vi "display queue.vi"(7 "Action":T1=enum."Enqueue", 8 "error in (no error)":errorcluster, 9 "max queue size (-1, unlimited)":i32=1, 10 "time out":i32=100, 11 "input data":u16[](array[numeric])) -> (0 "error out":errorcluster, 1 "timed out?":bool, 2 "Empty?":bool, 3 "output data":u16[](array[numeric]), 5 "# elements in queue":i32)   [LabVIEW 2018]
uses:
  Controls/Queue Manager Actions.ctl
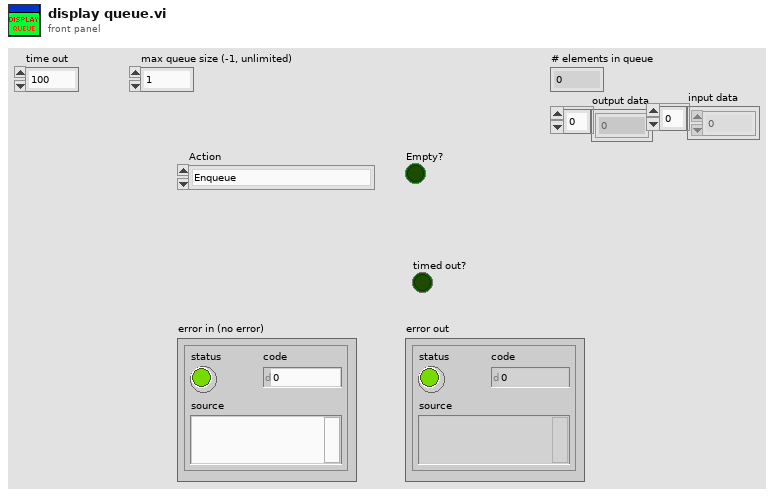
[diagram p1: front panel]
types:
  T1 = typedef "Queue Manager Actions.ctl" = enum16{"Init", "Enqueue", "Enqueue All", "Preview Queue", "Dequeue", "Get Status", "Flush Queue", "Flush All Queues", "Release All Queues", "Release Queue", "Enqueue at Opposite End"}
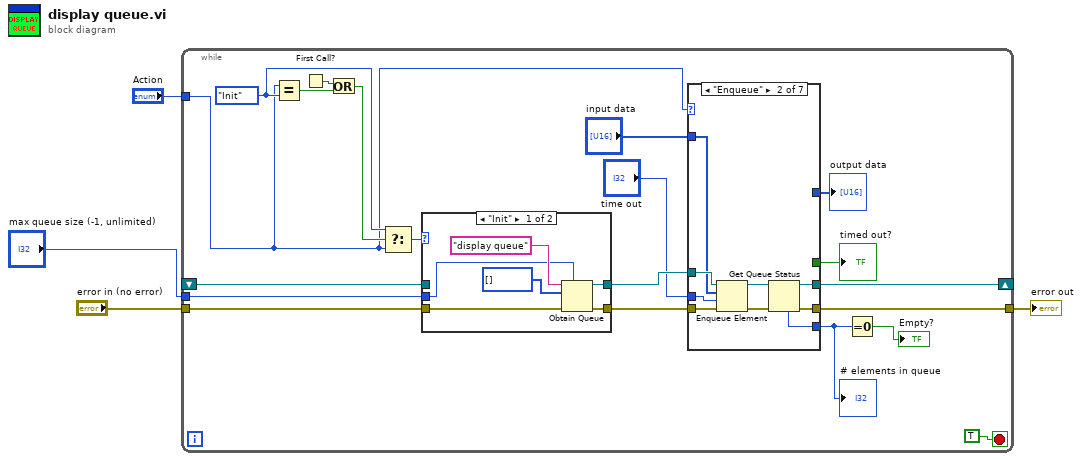
[diagram p0: block diagram]
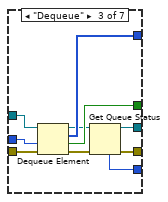
[diagram p3: hidden frame]
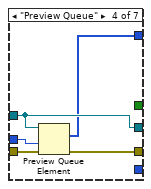
[diagram p4: hidden frame]
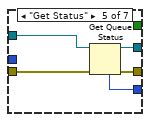
[diagram p5: hidden frame]
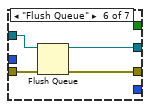
[diagram p6: hidden frame]
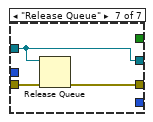
[diagram p7: hidden frame]
diagram:
  n1 = while {
    tunnel: "Action" -> [w12]
    tunnel: "error in (no error)" -> [w19]
    tunnel: [w18] -> w2
    shift-right: [w14] -> _
    shift-left: _ -> [w13]
    tunnel: "max queue size (-1, unlimited)" -> [w7]
    stop <- TRUE stop-if-true
    w21 = Queue_Manager_Actions."Init"
    n2 = Equal?(x=w12, y=w21) -> (x = y?=w23:bool)
    n3 = First Call?() -> (First Call?: T/F=w24:bool)
    n4 = Or(x=w24, y=w23) -> (x .or. y?=w22:bool)
    n5 = Select(t=w21, s=w22, f=w12) -> (s? t:f=w20:T1)
    n6 = case shown="\"Init\"" w20 {
      tunnel: [w68 w69] -> w16
      tunnel: w19 -> [w67 w70]
      tunnel: [w66 w70] -> w17
      tunnel: w13 -> [_ w69]
      tunnel: w7 -> [w63 _]
      frame "Init" {
        n7 = Obtain Queue(max queue size (-1, unlimited)=w63, name (unnamed)="display queue" ("queue name"), element data type=u16[] [], error in (no error)=w67) -> (queue out=w68:refnum<queue>, error out=w66:errorcluster)  [unwired: 1 in, 1 out]
      }
      frame "Enqueue", Default {
      }
    }
    n8 = case shown="\"Enqueue\"" w12 {
      tunnel: w16 -> [w25 w33 w43 w47 w53 w57 w60]
      tunnel: [w26 w29 w39 w49 w54 w58 w61] -> w18
      tunnel: w17 -> [w26 w35 w45 w50 w55 w59 w62]
      tunnel: [w25 w31 w38 w47 w52 w56 w60] -> w14
      tunnel: "time out" -> [_ w34 w44 w48 _ _ _]
      tunnel: [_ w28 w36 _ w51 _ _] -> w10
      tunnel: [_ _ w42 w46 _ _ _] -> w6
      tunnel: [_ _ w41 _ _ _ _] -> w9
      tunnel: "input data" -> [_ w27 _ _ _ _ _]
      frame "Init", Default {
      }
      frame "Enqueue" {
        n9 = Enqueue Element(queue=w33, element=w27, timeout in ms (-1)=w34, error in (no error)=w35) -> (queue out=w32:refnum<queue>, error out=w30:errorcluster)  [unwired: 1 out]
        n10 = Get Queue Status(queue=w32, error in (no error)=w30) -> (queue out=w31:refnum<queue>, error out=w29:errorcluster, # elements in queue=w28:i32)  [unwired: 1 in, 5 out]
      }
      frame "Dequeue" {
        n11 = Dequeue Element(queue=w43, timeout in ms (-1)=w44, error in (no error)=w45) -> (queue out=w37:refnum<queue>, element=w42:u16[], timed out?=w41:bool, error out=w40:errorcluster)
        n12 = Get Queue Status(queue=w37, error in (no error)=w40) -> (queue out=w38:refnum<queue>, error out=w39:errorcluster, # elements in queue=w36:i32)  [unwired: 1 in, 5 out]
      }
      frame "Preview Queue" {
        n13 = Preview Queue Element(queue=w47, timeout in ms (-1)=w48, error in (no error)=w50) -> (element=w46:u16[], error out=w49:errorcluster)  [unwired: 2 out]
      }
      frame "Get Status" {
        n14 = Get Queue Status(queue=w53, error in (no error)=w55) -> (queue out=w52:refnum<queue>, error out=w54:errorcluster, # elements in queue=w51:i32)  [unwired: 1 in, 5 out]
      }
      frame "Flush Queue" {
        n15 = Flush Queue(queue=w57, error in (no error)=w59) -> (queue out=w56:refnum<queue>, error out=w58:errorcluster)  [unwired: 1 out]
      }
      frame "Release Queue" {
        n16 = Release Queue(queue=w60, error in (no error)=w62) -> (error out=w61:errorcluster)  [unwired: 1 in, 2 out]
      }
    }
    "timed out?" <- w9
    "# elements in queue" <- w10
    "output data" <- w6
    n17 = Equal To 0?(x=w10) -> (x = 0?=→"Empty?":bool)
  }
  "error out" <- w2
